vi "test27-MappingRelationshipByLocalRegistration_WithoutSubcriberName.vi"(8 "error in (no error)":errorcluster, 11 "TestCase in":refnum<class "testcase-CSMBroadcast.lvclass">) -> (0 "error out":errorcluster, 3 "TestCase out":refnum<class "testcase-CSMBroadcast.lvclass">)   [LabVIEW 2017, in "testcase-CSMBroadcast.lvclass"]
uses:
  testcase-CSMBroadcast.lvclass
  47fe1622-87c8-40c1-b9cf-9bbb5cd90bb5.vi
  <vilib>/addons/_JKI Toolkits/VI Tester/TestCase.llb/TestCase.lvclass
  src/user.lib/_NEVSTOP/Communicable State Machine(CSM)/Communicable State Machine.lvlib
  CSM/CSM-Testcase.lvlib
  C:/Program Files (x86)/National Instruments/LabVIEW 2017/vi.lib/addons/_JKI Toolkits/VI Tester/TestCase.llb/TestCase.lvclass
panel:
  out "Loop Count":i32
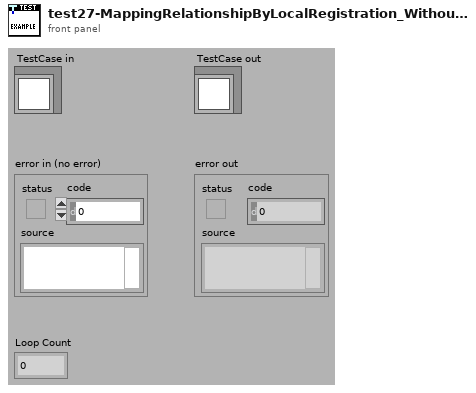
[diagram p1: front panel]
types:
  T1 = cluster{"Status":string, "Source CSM":string, "Target CSM":string, "Target API":string}[]
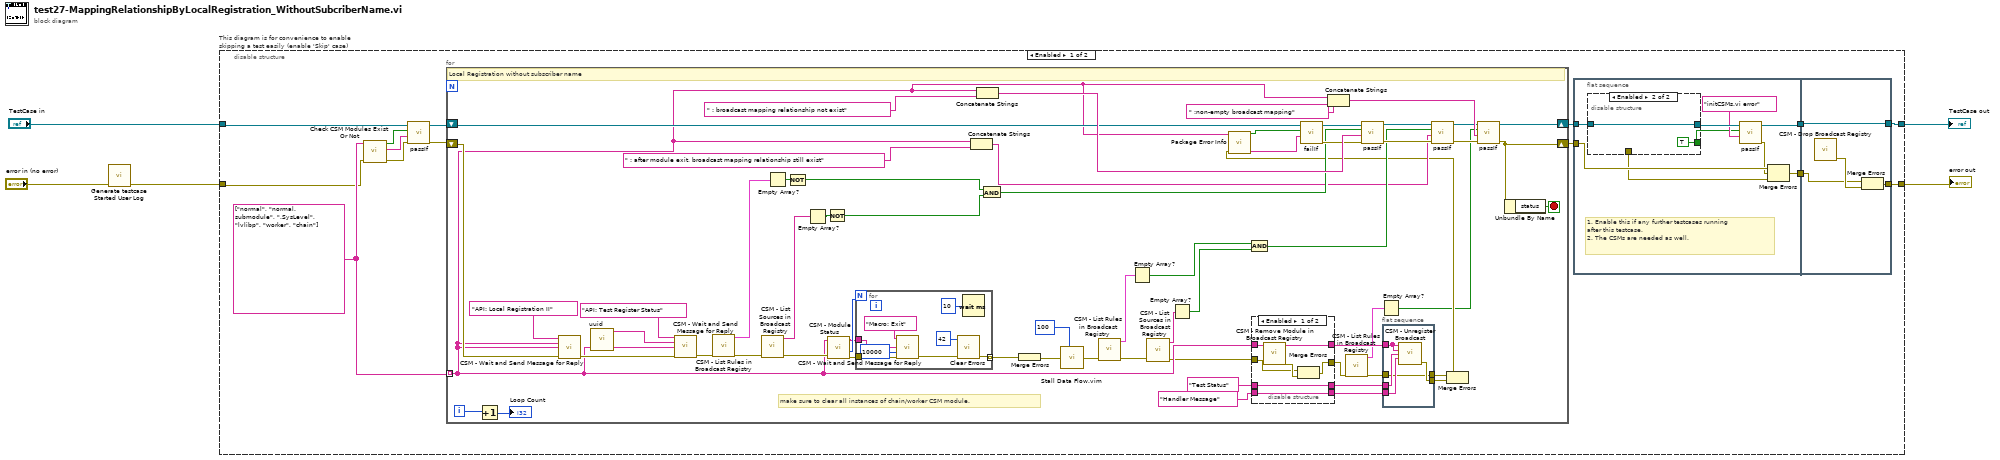
[diagram p0: block diagram]
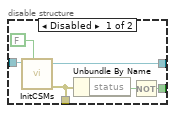
[diagram p2: hidden frame]
diagram:
  n1 = call "Generate testcase Started User Log.vi"("Error In"="error in (no error)") -> ("error out"=w1:errorcluster)  [unwired: 10 in]
  n2 = disable-structure "This diagram is for convenience to enable skipping a test easily (enable 'Skip' case)" shown="Enabled" {
    disable-tunnel: "TestCase in" -> [w15 w130]
    disable-tunnel: [w8 w128] -> w2
    disable-tunnel: [w6 w129] -> w4
    disable-tunnel: w1 -> [w14 w127]
    frame Enabled {
      w16 = string[] ["normal", "normal.submodule", ".SysLevel", "lvlibp", "worker", "chain"]
      n3 = call "Check CSM Modules Exist Or Not.vi"("error in"=w14, "CSM names in"=w16) -> ("error out"=w17:errorcluster, "Debug string"=w18:string, "All Modules Exist?"=w19:bool)  [unwired: 7 in]
      n4 = call-dynamic "passIf.vi"("error in (no error)"=w17, "message (\"\")"=w18, "pass"=w19, "TestCase in"=w15) -> ("error out"=w12:errorcluster, "TestCase out"=w13:refnum<class "testcase-CSMBroadcast.lvclass">)  [unwired: 6 in]
      n5 = for {
        tunnel: w16 -> [w47] mode=indexing
        shift-right: [w86] -> w9
        shift-left: w13 -> [w70]
        shift-right: [w87] -> w7
        shift-left: w12 -> [w85]
        i -> [w93]
        stop <- w96 stop-if-true
        # "make sure to clear all instances of chain/worker CSM module."
        # "Local Registration without subscriber name"
        n6 = Increment(x=w93) -> (x+1=→"Loop Count":i32)
        n7 = call "CSM - Wait and Send Message for Reply.vi"("State"="API: Local Registration II", "Arguments (\"\")"=w47, "Target Module"=w47, "Error In (No Error)"=w85) -> ("error out"=w101:errorcluster)  [unwired: 8 in, 3 out]
        n8 = call "uuid.vi"() -> ("UUID"=w99:string)  [unwired: 11 in]
        n9 = call "CSM - Wait and Send Message for Reply.vi"("State"="API: Test Register Status", "Arguments (\"\")"=w99, "Target Module"=w47, "Error In (No Error)"=w101) -> ("error out"=w98:errorcluster)  [unwired: 8 in, 3 out]
        n10 = call "CSM - List Rules in Broadcast Registry.vi"("error in (no error)"=w98) -> ("error out"=w95:errorcluster, "Rule Entries"=w91:T1)  [unwired: 8 in, 1 out]
        n11 = call "CSM - List Sources in Broadcast Registry.vi"("error in (no error)"=w95) -> ("error out"=w82:errorcluster, "Broadcast Names"=w88:string[])  [unwired: 9 in]
        n12 = Empty Array?(array=w91) -> (empty?=w90:bool)
        n13 = Not(x=w90) -> (.not. x?=w66:bool)
        n14 = Empty Array?(array=w88) -> (empty?=w89:bool)
        n15 = Not(x=w89) -> (.not. x?=w65:bool)
        n16 = call "CSM - Module Status.vi"("Error In"=w82, "CSM Name"=w47) -> ("error out"=w81:errorcluster, "#Nodes"=w84:i32, "CSM Name (Dup)"=w83:string)  [unwired: 5 in, 2 out]
        n17 = for {
          N: w84 -> [_]
          tunnel: [w121] -> w97 mode=indexing
          tunnel: w83 -> [w125]
          tunnel: w81 -> [w124]
          n18 = call "CSM - Wait and Send Message for Reply.vi"("State"="Macro: Exit", "Target Module"=w125, "Wait (5000ms)"=10000, "Error In (No Error)"=w124) -> ("error out"=w122:errorcluster)  [unwired: 8 in, 3 out]
          n19 = call <vilib>:"Clear Errors.vi"("error in (no error)"=w122, "specific error code to clear (0: all)"=42) -> ("error out"=w121:errorcluster)  [unwired: 4 in, 1 out]
          n20 = Wait (ms)(milliseconds to wait=u32 10) -> ()  [unwired: 1 out]
        }
        n21 = Concatenate Strings(w47, " : after module exit, broadcast mapping relationship still exist" ("string")) -> (w55:string)
        n22 = Concatenate Strings(w47, " : broadcast mapping relationship not exist" ("string")) -> (w77:string)
        n23 = And(x=w66, y=w65) -> (x .and. y?=w62:bool)
        n24 = Merge Errors(w97) -> (w76:errorcluster)
        n25 = call "Stall Data Flow.vim"("value in"=w76, "milliseconds to wait"=u32 100) -> ("value out"=w75:errorcluster)  [unwired: 1 out]
        n26 = call "CSM - List Rules in Broadcast Registry.vi"("error in (no error)"=w75) -> ("error out"=w94:errorcluster, "Rule Entries"=w68:T1)  [unwired: 8 in, 1 out]
        n27 = Empty Array?(array=w68) -> (empty?=w64:bool)
        n28 = call "CSM - List Sources in Broadcast Registry.vi"("error in (no error)"=w94) -> ("error out"=w46:errorcluster, "Broadcast Names"=w67:string[])  [unwired: 9 in]
        n29 = Empty Array?(array=w67) -> (empty?=w63:bool)
        n30 = And(x=w64, y=w63) -> (x .and. y?=w57:bool)
        n31 = disable-structure shown="Enabled" {
          disable-tunnel: w46 -> [w108 w117]
          disable-tunnel: [w112 w117] -> w53
          disable-tunnel: w47 -> [w113 w118]
          disable-tunnel: "Test Status" ("Status") -> [w110 w116]
          disable-tunnel: "Handler Message" ("Response Message (If \"\", Same as Source Message)") -> [w109 w115]
          disable-tunnel: [w111 w118] -> w54
          disable-tunnel: [w110 w116] -> w52
          disable-tunnel: [w109 w115] -> w51
          frame Enabled {
            n32 = call "CSM - Remove Module in Broadcast Registry.vi"("CSM Name"=w113) -> ("CSM Name (Dup)"=w111:string, "error out"=w114:errorcluster)  [unwired: 13 in]
            n33 = Merge Errors(w108, w114) -> (w112:errorcluster)
          }
          frame Disabled {
          }
        }
        n34 = Concatenate Strings(w47, " :non-empty broadcast mapping" ("string")) -> (w78:string)
        n35 = call "CSM - List Rules in Broadcast Registry.vi"("error in (no error)"=w53) -> ("error out"=w49:errorcluster, "Rule Entries"=w42:T1)  [unwired: 8 in, 1 out]
        n36 = Empty Array?(array=w42) -> (empty?=w41:bool)
        n37 = flat-sequence {
          tunnel: w54 -> [w107]
          tunnel: w52 -> [w106]
          tunnel: w51 -> [w105]
          tunnel: [w104] -> w50
          tunnel: w49 -> [w103]
          tunnel: [w103] -> w48
          frame #0 {
            n38 = call "CSM - Unregister Broadcast.vi"("CSM Name(Empty for Broadcast Event)"=w107, "Source CSM Name (* as Default)"=w107, "Trigger"=w106, "API (\"*\" as Default)"=w105) -> ("error out"=w104:errorcluster)  [unwired: 10 in, 1 out]
          }
        }
        n39 = Merge Errors(w48, w50) -> (w45:errorcluster)
        n40 = call "Package Error Info.vi"("error in"=w45, "String in"=w47) -> ("packed error info out"=w73:string, "error status"=w72:bool)  [unwired: 8 in]
        n41 = call-dynamic "failIf.vi"("message (\"\")"=w73, "fail"=w72, "TestCase in"=w70) -> ("error out"=w71:errorcluster, "TestCase out"=w69:refnum<class "testcase-CSMBroadcast.lvclass">)  [unwired: 7 in]
        n42 = call-dynamic "passIf.vi"("error in (no error)"=w71, "message (\"\")"=w77, "pass"=w62, "TestCase in"=w69) -> ("error out"=w59:errorcluster, "TestCase out"=w61:refnum<class "testcase-CSMBroadcast.lvclass">)  [unwired: 6 in]
        n43 = call-dynamic "passIf.vi"("error in (no error)"=w59, "message (\"\")"=w55, "pass"=w57, "TestCase in"=w61) -> ("error out"=w58:errorcluster, "TestCase out"=w60:refnum<class "testcase-CSMBroadcast.lvclass">)  [unwired: 6 in]
        n44 = call-dynamic "passIf.vi"("error in (no error)"=w58, "message (\"\")"=w78, "pass"=w41, "TestCase in"=w60) -> ("error out"=w87:errorcluster, "TestCase out"=w86:refnum<class "testcase-CSMBroadcast.lvclass">)  [unwired: 6 in]
        n45 = Unbundle By Name(w87) -> ("status"=w96:bool)
      }
      n46 = flat-sequence {
        tunnel: w9 -> [w28]
        tunnel: [w26] -> w11
        tunnel: w7 -> [w24]
        tunnel: [w21] -> w10
        tunnel: w11 -> [w39]
        tunnel: [w39] -> w8
        tunnel: [w38] -> w6
        tunnel: w10 -> [w37]
        frame #0 {
          # "1. Enable this if any further testcases running\nafter this testcase.\n2. The CSMs are needed as well."
          n47 = disable-structure shown="Enabled" {
            disable-tunnel: w28 -> [w34 w36]
            disable-tunnel: [w32 w36] -> w27
            disable-tunnel: [w30 _] -> w22
            disable-tunnel: [w29 TRUE ("pass")] -> w20
            frame Disabled {
              n48 = call "InitCSMs.vi"("Enable building lvlibp?"=FALSE, "testcase-CSMStatus in"=w34) -> ("error out"=w30:errorcluster, "testcase-CSMStatus out"=w32:refnum<class "testcase-CSMBroadcast.lvclass">)  [unwired: 8 in]
              n49 = Unbundle By Name(w30) -> ("status"=w31:bool)
              n50 = Not(x=w31) -> (.not. x?=w29:bool)
            }
            frame Enabled {
            }
          }
          n51 = call-dynamic "passIf.vi"("message (\"\")"="initCSMs.vi error" ("message (\"\")"), "pass"=w20, "TestCase in"=w27) -> ("error out"=w23:errorcluster, "TestCase out"=w26:refnum<class "testcase-CSMBroadcast.lvclass">)  [unwired: 7 in]
          n52 = Merge Errors(w24, w23, w22) -> (w21:errorcluster)
        }
        frame #1 {
          n53 = call "CSM - Drop Broadcast Registry.vi"() -> ("error out"=w40:errorcluster)  [unwired: 15 in]
          n54 = Merge Errors(w37, w40) -> (w38:errorcluster)
        }
      }
    }
    frame Disabled {
      # "skip test result while test is under development"
      n55 = call <vilib>:"skip.vi"("error in (no error)"=w127, "TestCase in"=w130) -> ("error out"=w129:errorcluster, "TestCase out"=w128:refnum<class "testcase-CSMBroadcast.lvclass">)  [unwired: 8 in]
    }
  }
  "error out" <- w4
  "TestCase out" <- w2
